vi "Nfocus driver.vi"(5 "error in":errorcluster, 8 "Refs In":T1) -> (0 "error out":errorcluster)   [LabVIEW 2016]
panel:
  out "Running":bool
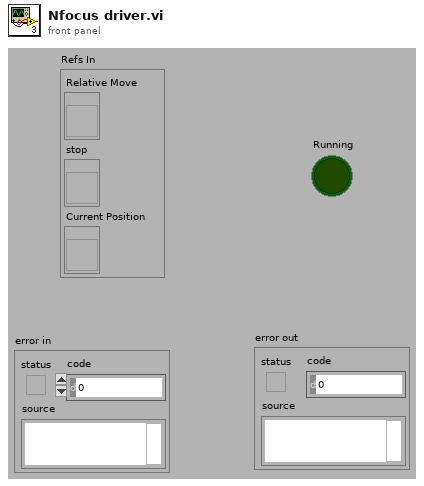
[diagram p1: front panel]
types:
  T1 = cluster{"Relative Move":refnum<vi>, "stop":refnum<vi>, "Current Position":refnum<vi>}
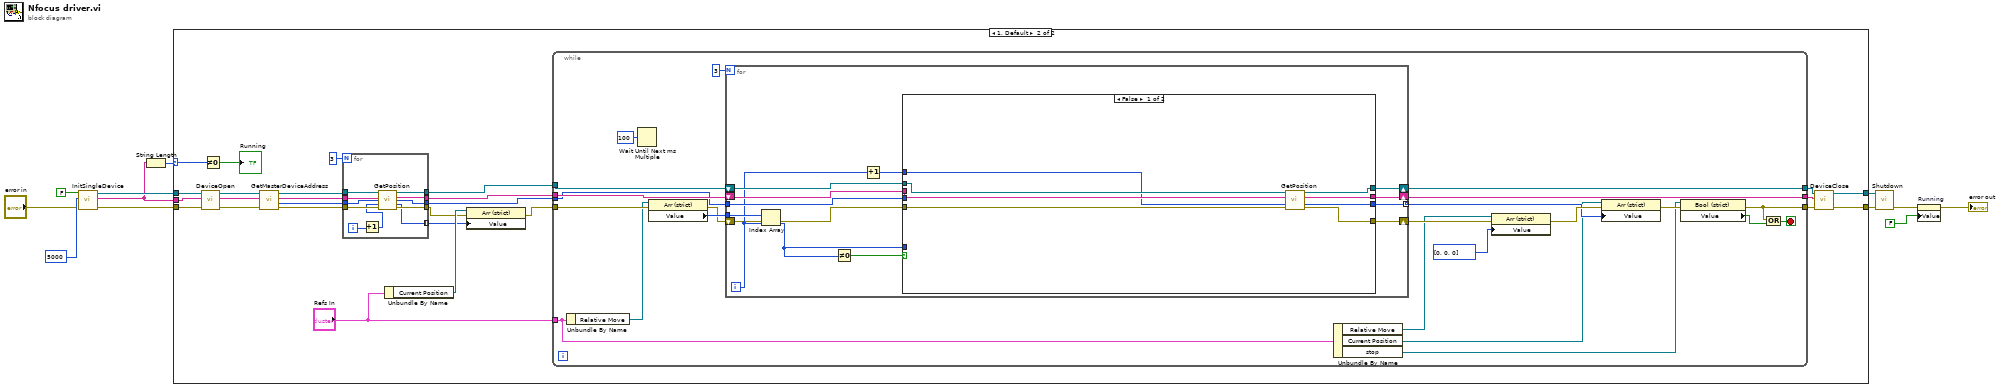
[diagram p0: block diagram]
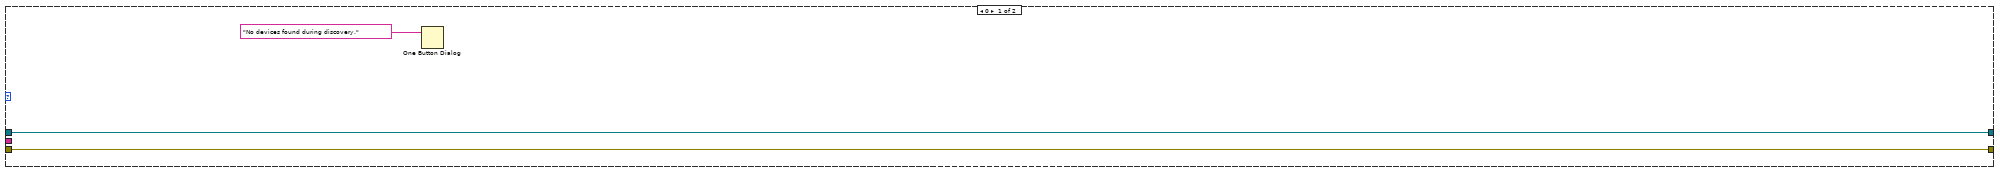
[diagram p2: hidden frame]
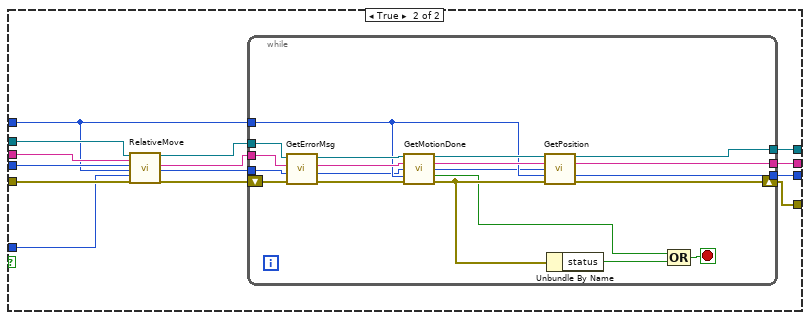
[diagram p3: hidden frame]
diagram:
  n1 = call "InitSingleDevice.vi"("error in (no error)"="error in", "msecDelayForDiscovery"=5000, "logging"=FALSE) -> ("error out"=w5:errorcluster, "DeviceKey Out"=w6:string, "CmdLib Out"=w8:refnum<k24>)  [unwired: 2 in]
  n2 = String Length(string=w6) -> (length=w7:i32)
  n3 = case shown="1, Default" w7 {
    selector: w7 -> [_ w30]
    tunnel: [w14 w31] -> w10
    tunnel: [w13 w33] -> w9
    tunnel: w8 -> [w14 w37]
    tunnel: w6 -> [_ w39]
    tunnel: w5 -> [w13 w41]
    frame 0 {
      n4 = One Button Dialog(message="No devices found during discovery.") -> ()  [unwired: 1 in, 1 out]
    }
    frame 1, Default {
      n5 = call "DeviceOpen.vi"("error in (no error)"=w41, "DeviceKey In"=w39, "CmdLib In"=w37) -> ("error out"=w40:errorcluster, "DeviceKey Out"=w38:string, "CmdLib Out"=w36:refnum<k24>)  [unwired: 2 in]
      n6 = Not Equal To 0?(x=w30) -> (x != 0?=→"Running":bool)
      n7 = call "GetMasterDeviceAddress.vi"("error in (no error)"=w40, "DeviceKey In"=w38, "CmdLib In"=w36) -> ("error out"=w28:errorcluster, "Device Address"=w27:i32, "DeviceKey Out"=w26:string, "CmdLib Out"=w25:refnum<k24>)  [unwired: 1 in]
      n8 = for {
        N: 3 -> [_]
        tunnel: w25 -> [w49]
        tunnel: [w48] -> w24
        tunnel: w26 -> [w50]
        tunnel: [w47] -> w23
        tunnel: w27 -> [w51]
        tunnel: [w46] -> w22
        tunnel: w28 -> [w52]
        tunnel: [w45] -> w18
        tunnel: [w42] -> w19 mode=indexing
        i -> [w44]
        n9 = Increment(x=w44) -> (x+1=w43:i32)
        n10 = call "GetPosition.vi"("CmdLib In"=w49, "DeviceKey In"=w50, "Device Address In"=w51, "Motor"=w43, "error in (no error)"=w52) -> ("CmdLib Out"=w48:refnum<k24>, "DeviceKey Out"=w47:string, "Device Address Out"=w46:i32, "Position"=w42:i32, "error out"=w45:errorcluster)  [unwired: 6 in]
      }
      n11 = Unbundle By Name("Refs In") -> ("Current Position"=w20:refnum<vi>)
      n12 = property class="Arr (strict)"(reference=w20, error in=w18, "Value"=w19) -> (error out=w17:errorcluster)  [unwired: 1 out]
      n13 = while {
        tunnel: w22 -> [w65]
        tunnel: w24 -> [w67]
        tunnel: [w74] -> w32
        tunnel: w17 -> [w69]
        tunnel: [w72] -> w34
        tunnel: w23 -> [w66]
        tunnel: [w75] -> w35
        tunnel: "Refs In" -> [w58]
        stop <- w73 stop-if-true
        n14 = Unbundle By Name(w58) -> ("Relative Move"=w63:refnum<vi>)
        n15 = Wait Until Next ms Multiple(millisecond multiple=u32 100) -> ()  [unwired: 1 out]
        n16 = property class="Arr (strict)"(reference=w63, error in=w69) -> (error out=w68:errorcluster, "Value"=w70:i32[])  [unwired: 1 out]
        n17 = for {
          N: 3 -> [_]
          tunnel: w70 -> [w85]
          shift-right: [w80] -> w64
          shift-left: w68 -> [w84]
          shift-right: [w87] -> w74
          shift-left: w67 -> [w83]
          shift-right: [w88] -> w75
          shift-left: w66 -> [w82]
          tunnel: w65 -> [w81]
          tunnel: [w79] -> w59 mode=indexing
          i -> [w77]
          n18 = Index Array(array=w85, index=w77) -> (element=w78:i32)
          n19 = Not Equal To 0?(x=w78) -> (x != 0?=w86:bool)
          n20 = Increment(x=w77) -> (x+1=w76:i32)
          n21 = case shown="False" w86 {
            tunnel: w81 -> [_ w110]
            tunnel: w83 -> [w96 w109]
            tunnel: w82 -> [w95 w108]
            tunnel: [w92 w107] -> w88
            tunnel: [w91 w106] -> w87
            tunnel: w84 -> [w94 w105]
            tunnel: [w93 w104] -> w80
            tunnel: [w90 w99] -> w79
            tunnel: w78 -> [_ w98]
            tunnel: w76 -> [w89 w97]
            frame False {
              n22 = call "GetPosition.vi"("CmdLib In"=w96, "DeviceKey In"=w95, "Motor"=w89, "error in (no error)"=w94) -> ("CmdLib Out"=w91:refnum<k24>, "DeviceKey Out"=w92:string, "Position"=w90:i32, "error out"=w93:errorcluster)  [unwired: 7 in, 1 out]
            }
            frame True {
              n23 = call "RelativeMove.vi"("CmdLib In"=w109, "DeviceKey In"=w108, "Device Address In"=w110, "Motor"=w97, "Relative Steps"=w98, "error in (no error)"=w105) -> ("CmdLib Out"=w103:refnum<k24>, "DeviceKey Out"=w102:string, "Device Address Out"=w100:i32, "error out"=w101:errorcluster)  [unwired: 10 in]
              n24 = while {
                tunnel: w97 -> [w126]
                tunnel: w103 -> [w125]
                tunnel: w102 -> [w124]
                tunnel: [w119] -> w106
                tunnel: w100 -> [w118]
                shift-right: [w120] -> w104
                shift-left: w101 -> [w123]
                tunnel: [w115] -> w107
                tunnel: [w111] -> w99
                stop <- w114 stop-if-true
                n25 = call "GetErrorMsg.vi"("error in (no error)"=w123, "Device Address In"=w118, "DeviceKey In"=w124, "CmdLib In"=w125) -> ("error out"=w122:errorcluster, "Device Address Out"=w117:i32, "DeviceKey Out"=w128:string, "CmdLib Out"=w127:refnum<k24>)
                n26 = call "GetMotionDone.vi"("CmdLib In"=w127, "DeviceKey In"=w128, "Device Address In"=w117, "Motor"=w126, "error in (no error)"=w122) -> ("CmdLib Out"=w129:refnum<k24>, "DeviceKey Out"=w130:string, "Device Address Out"=w116:i32, "Is Motion Done"=w113:bool, "error out"=w121:errorcluster)  [unwired: 6 in]
                n27 = call "GetPosition.vi"("CmdLib In"=w129, "DeviceKey In"=w130, "Device Address In"=w116, "Motor"=w126, "error in (no error)"=w121) -> ("CmdLib Out"=w119:refnum<k24>, "DeviceKey Out"=w115:string, "Position"=w111:i32, "error out"=w120:errorcluster)  [unwired: 6 in, 1 out]
                n28 = Unbundle By Name(w121) -> ("status"=w112:bool)
                n29 = Compound Arithmetic op=OR(w113, w112) -> (w114:bool)
              }
            }
          }
        }
        n30 = Unbundle By Name(w58) -> ("Relative Move"=w54:refnum<vi>, "Current Position"=w57:refnum<vi>, "stop"=w56:refnum<vi>)
        n31 = property class="Arr (strict)"(reference=w54, error in=w64, "Value"=i32[] [0, 0, 0]) -> (error out=w61:errorcluster)  [unwired: 1 out]
        n32 = property class="Arr (strict)"(reference=w57, error in=w61, "Value"=w59) -> (error out=w60:errorcluster)  [unwired: 1 out]
        n33 = property on="Property Node" class="Bool (strict)"(reference=w56, error in=w60) -> (error out=w72:errorcluster, "Value"=w71:bool)  [unwired: 1 out]
        n34 = Compound Arithmetic op=OR(w72, w71) -> (w73:bool)
      }
      n35 = call "DeviceClose.vi"("error in (no error)"=w34, "DeviceKey In"=w35, "CmdLib In"=w32) -> ("error out"=w33:errorcluster, "CmdLib Out"=w31:refnum<k24>)  [unwired: 2 in, 1 out]
    }
  }
  n36 = call "Shutdown.vi"("error in (no error)"=w9, "CmdLib In"=w10) -> ("error out"=w3:errorcluster)  [unwired: 4 in, 1 out]
  n37 = property on="Running" class="Bool (strict)"(error in=w3, "Value"=FALSE ("Boolean")) -> (error out=→"error out":errorcluster)  [unwired: 1 in, 1 out]
